vi "PostCopyScripting.vi"(10 "MetaDataObj":refnum<class "MetaDataObj.lvclass">, 11 "User Project":refnum<vi>) -> ()   [LabVIEW 2013, in "FixedChannelTBModuleDecideFeatures.lvclass"]
uses:
  FixedChannelTBModuleDecideFeatures.lvclass
  <resource>/dialog/NewProjectWizard/MetaDataObj/MetaDataObj.lvclass
  <vilib>/NI/Tag Bus Data Framework/control module/script/Controls/processing script control.ctl
  <vilib>/NI/Tag Bus Data Framework/control module/script/Controls/output script control.ctl
  <vilib>/NI/Tag Bus Data Framework/control module/script/Controls/input script control.ctl
  FixedChannelTBModuleDecideFeatures.lvclass/FixedChannelTBModuleDecideFeatures.ctl
  Read component name.vi
  Read Channel Specification.vi
  <vilib>/NI/Tag Bus Data Framework/control module/script/control module data interface generator.lvlib
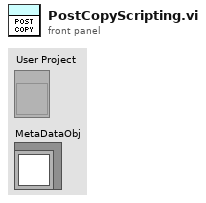
[diagram p1: front panel]
types:
  T1 = typedef "control module data interface generator.lvlib/input script control.ctl" = cluster{"enable?":bool, "Data Interface VI (blank=input to tag bus.vi)":string, "reverse?":bool, "Reverse Interface VI (blank=input from tag bus.vi)":string}
  T2 = typedef "control module data interface generator.lvlib/output script control.ctl" = cluster{"enable?":bool, "Data Interface VI (blank=tag bus to outputs.vi)":string, "Reverse Interface VI (blank=tag bus from outputs.vi)":string, "reverse?":bool}
  T3 = typedef "control module data interface generator.lvlib/processing script control.ctl" = cluster{"param?":bool, "Parameter Data Interface VI (blank=tag bus to parameters.vi)":string, "Result Data Interface VI (blank=results to tag bus.vi)":string, "reverse param?":bool, "Rev. Result Interface VI (blank=results from tag bus.vi)":string, "Rev. Parameter Interface VI (blank=tag bus from parameters.vi)":string, "result?":bool, "reverse result?":bool}
  T4 = typedef "FixedChannelTBModuleDecideFeatures.lvclass/channel configuration.ctl" = cluster{"Name":string, "channel classification":T5, "data type":T6}
  T5 = typedef "TBM channel.lvclass/channel classification.ctl" = enum16{"input data", "output data", "processing parameter", "processing result"}
  T6 = typedef "tag bus.lvlib/tag descriptor.lvclass/Data Type.ctl" = enum16{"Double", "Single", "I64", "I32", "I16", "I8", "U64", "U32", "U16", "U8", "Boolean", "String", "Array of Double", "Array of Single", "Array of I64", "Array of I32", "Array of I16", "Array of I8", "Array of U64", "Array of U32", "Array of U16", "Array of U8", "Array of Boolean", "Array of String"}
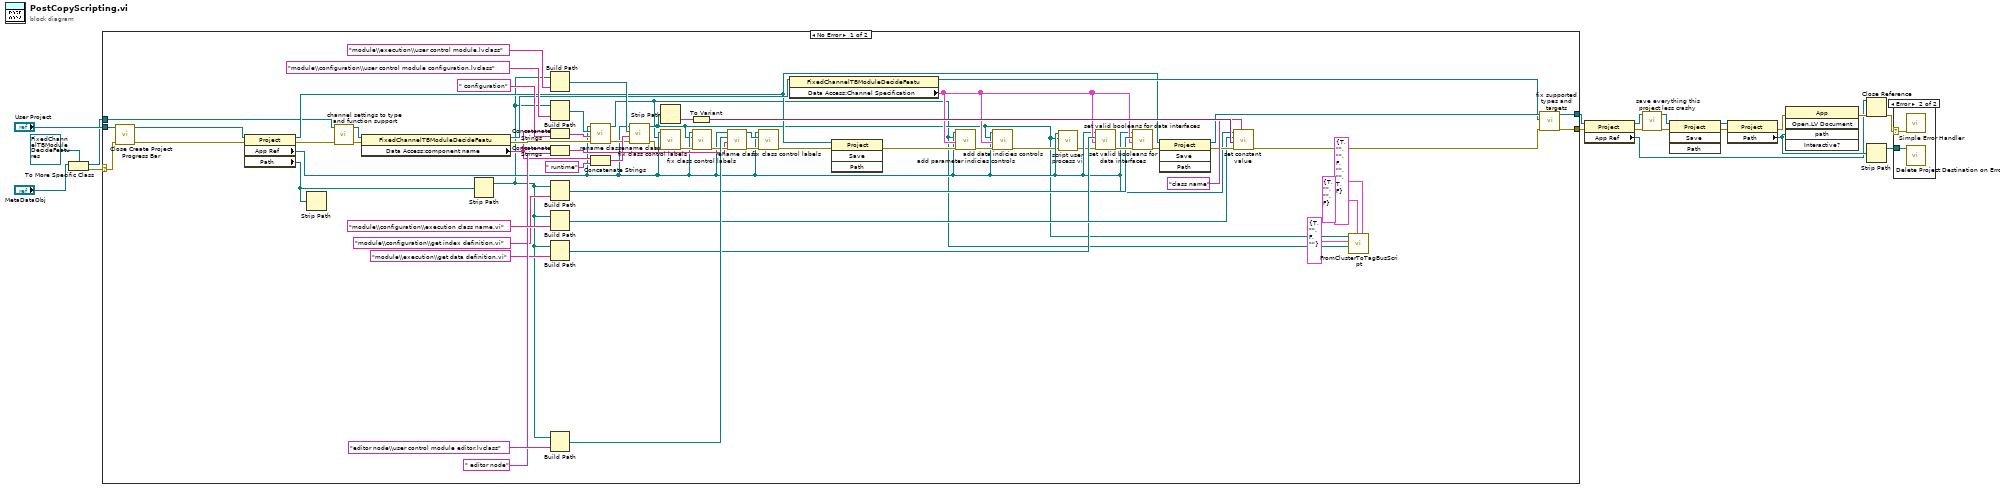
[diagram p0: block diagram]
diagram:
  n1 = To More Specific Class(target class=refnum<class "FixedChannelTBModuleDecideFeatures.lvclass"> refnum ("DecideProjectFeatures.lvclass"), reference="MetaDataObj") -> (specific class reference=w10:refnum<class "FixedChannelTBModuleDecideFeatures.lvclass">, error out=w17:errorcluster)  [unwired: 1 in]
  n2 = case shown="No Error" w17 {
    selector: w17 -> [w38 w81]
    tunnel: [w60 w82] -> w2
    tunnel: "User Project" -> [w39 w82]
    tunnel: [w61 w81] -> w1
    tunnel: w10 -> [w45 _]
    frame No Error {
      n3 = call <resource>:"Close Create Project Progress Bar.vi"("error in (no error)"=w38, "Project"=w39) -> ("error out"=w37:errorcluster, "dup Project"=w36:refnum<vi>)  [unwired: 8 in]
      n4 = property class="Project"(reference=w36, error in=w37) -> (reference out=w50:refnum<vi>, error out=w44:errorcluster, "App Ref"=w28:refnum<vi>, "Path"=w49:path)
      n5 = Strip Path(path=w49) -> ()  [unwired: 2 out]
      n6 = call "channel settings to type and function support.vi"("error in"=w44, "FixedChannelTBModuleDecideFeatures in"=w45) -> ("error out"=w47:errorcluster, "FixedChannelTBModuleDecideFeatures out"=w46:refnum<class "FixedChannelTBModuleDecideFeatures.lvclass">)  [unwired: 8 in]
      n7 = property class="FixedChannelTBModuleDecideFeatu"(reference=w46, error in=w47) -> (reference out=w76:refnum<class "FixedChannelTBModuleDecideFeatures.lvclass">, error out=w48:errorcluster, "Data Access:component name"=w41:string)
      n8 = Strip Path(path=w49) -> (stripped path=w26:path)  [unwired: 1 out]
      n9 = Build Path(base path=w26, name or relative path="module\\execution\\user control module.lvclass") -> (appended path=w78:path)
      n10 = Build Path(base path=w26, name or relative path="module\\configuration\\user control module configuration.lvclass") -> (appended path=w53:path)
      n11 = Concatenate Strings(w41, " configuration" ("string")) -> (w58:string)
      n12 = Concatenate Strings(w41, " editor node" ("string")) -> (w62:string)
      n13 = Build Path(base path=w26, name or relative path="module\\configuration\\get index definition.vi") -> (appended path=w30:path)
      n14 = Build Path(base path=w26, name or relative path="module\\configuration\\execution class name.vi") -> (appended path=w43:path)
      n15 = Build Path(base path=w26, name or relative path="module\\execution\\get data definition.vi") -> (appended path=w33:path)
      n16 = Build Path(base path=w26, name or relative path="editor node\\user control module editor.lvclass") -> (appended path=w67:path)
      n17 = call "rename class.vi"("error in"=w48, "new name"=w58, "class path"=w53, "Application in"=w28) -> ("error out"=w54:errorcluster, "New Library Path"=w23:path)  [unwired: 6 in]
      n18 = Concatenate Strings(w41, " runtime" ("string")) -> (w55:string)
      n19 = call "rename class.vi"("error in"=w54, "new name"=w55, "class path"=w78, "Application in"=w28) -> ("error out"=w70:errorcluster, "New Library Path"=w24:path)  [unwired: 6 in]
      n20 = Strip Path(path=w24) -> (name=w57:string)  [unwired: 1 out]
      n21 = call "fix class control labels.vi"("error in"=w70, "class to load"=w23, "Application in"=w28) -> ("error out"=w69:errorcluster)  [unwired: 8 in]
      n22 = To Variant(anything=w57) -> (Variant=w75:variant)
      n23 = call "fix class control labels.vi"("error in"=w69, "class to load"=w24, "Application in"=w28) -> ("error out"=w64:errorcluster)  [unwired: 8 in]
      n24 = call "rename class.vi"("error in"=w64, "new name"=w62, "class path"=w67, "Application in"=w28) -> ("error out"=w65:errorcluster, "New Library Path"=w66:path)  [unwired: 6 in]
      n25 = call "fix class control labels.vi"("error in"=w65, "class to load"=w66, "Application in"=w28) -> ("error out"=w40:errorcluster)  [unwired: 8 in]
      n26 = property class="FixedChannelTBModuleDecideFeatu"(reference=w76) -> (reference out=w52:refnum<class "FixedChannelTBModuleDecideFeatures.lvclass">, "Data Access:Channel Specification"=w29:T4[])  [unwired: 1 in, 1 out]
      n27 = invoke class="Project" method="Save"(reference=w50, error in=w40) -> (error out=w51:errorcluster)  [unwired: 2 in, 3 out]
      n28 = call "add parameter indicies controls.vi"("error in"=w51, "Channels to create"=w29, "cfg class path"=w23, "Application in"=w28) -> ("error out"=w42:errorcluster)  [unwired: 7 in]
      n29 = call "add data indicies controls.vi"("error in"=w42, "Channels to create"=w29, "runtime class path"=w24, "Application in"=w28) -> ("error out"=w25:errorcluster)  [unwired: 6 in, 1 out]
      n30 = call "script user process vi.vi"("error in"=w25, "runtime class path in"=w24, "Application in"=w28) -> ("error out"=w27:errorcluster)  [unwired: 8 in]
      n31 = call "set valid booleans for data interfaces.vi"("error in"=w27, "Channel Specification"=w29, "vi path"=w33, "Application in"=w28) -> ("error out"=w32:errorcluster)  [unwired: 7 in]
      n32 = call "set valid booleans for data interfaces.vi"("error in"=w32, "Channel Specification"=w29, "vi path"=w30, "Application in"=w28) -> ("error out"=w31:errorcluster)  [unwired: 7 in]
      n33 = invoke class="Project" method="Save"(reference=w50, error in=w31) -> (reference out=w71:refnum<vi>, error out=w72:errorcluster)  [unwired: 2 in, 2 out]
      n34 = call "set constant value.vi"("control name"="class name", "error in"=w72, "data to set"=w75, "vi path"=w43, "Application in"=w28) -> ("error out"=w59:errorcluster)  [unwired: 6 in]
      n35 = call <vilib>:"FromClusterToTagBusScript.vi"("process"=T3 {"param?"=TRUE, "Parameter Data Interface VI (blank=tag bus to parameters.vi)"="", "Result Data Interface VI (blank=results to tag bus.vi)"="", "reverse param?"=FALSE, "Rev. Result Interface VI (blank=results from tag bus.vi)"="", "Rev. Parameter Interface VI (blank=tag bus from parameters.vi)"="", "result?"=TRUE, "reverse result?"=FALSE}, "output"=T2 {"enable?"=TRUE, "Data Interface VI (blank=tag bus to outputs.vi)"="", "Reverse Interface VI (blank=tag bus from outputs.vi)"="", "reverse?"=FALSE}, "configuration class path"=w23, "input"=T1 {"enable?"=TRUE, "Data Interface VI (blank=input to tag bus.vi)"="", "reverse?"=FALSE, "Reverse Interface VI (blank=input from tag bus.vi)"=""}, "runtime class path"=w24) -> ()  [unwired: 6 in, 1 out]
      n36 = call "fix supported types and targets.vi"("error in"=w59, "DecideProjectFeatures in"=w52, "User Project in"=w71) -> ("error out"=w61:errorcluster, "User Project out"=w60:refnum<vi>)  [unwired: 7 in]
    }
    frame Error {
    }
  }
  n37 = property class="Project"(reference=w2, error in=w1) -> (reference out=w7:refnum<vi>, error out=w8:errorcluster, "App Ref"=w6:refnum<vi>)
  n38 = call "save everything this project less crashy.vi"("error in"=w8, "Project in"=w7) -> ("error out"=w3:errorcluster, "Project out"=w9:refnum<vi>)  [unwired: 8 in]
  n39 = invoke class="Project" method="Save"(reference=w9, error in=w3) -> (reference out=w13:refnum<vi>, error out=w14:errorcluster)  [unwired: 2 in, 2 out]
  n40 = property class="Project"(reference=w13, error in=w14) -> (error out=w16:errorcluster, "Path"=w11:path)  [unwired: 1 out]
  n41 = invoke class="App" method="Open.LV Document"(error in=w16, "path"=w11) -> (error out=w15:errorcluster)  [unwired: 3 in, 4 out]
  n42 = Close Reference(reference=w6, error in (no error)=w15) -> (error out=w5:errorcluster)
  n43 = Strip Path(path=w11) -> (stripped path=w4:path)  [unwired: 1 out]
  n44 = case shown="Error" w5 {
    selector: w5 -> [_ w83]
    tunnel: w4 -> [_ w84]
    frame No Error {
    }
    frame Error {
      n45 = call <vilib>:"Simple Error Handler.vi"("error in (no error)"=w83) -> ()  [unwired: 4 in, 5 out]
      n46 = call <resource>:"Delete Project Destination on Error.vi"("Project Destination Root"=w84) -> ()  [unwired: 11 in]
    }
  }
